vi "DSB Modulation Demo (Baseband-Sine) - Basic.vi"() -> ()   [LabVIEW 2013]
uses:
  <vilib>/express/express analysis/Spectral/Block/exnSpectralBlock spectral measurements power poly.vi
  <vilib>/express/express analysis/Spectral/Block/exnSpectralBlock spectral measurements power DDT.vi
  <vilib>/express/express analysis/Spectral/XNode/ExpressSpectralMeasurementsBlockNode.xnode
panel:
  in  "WAV Sample Rate":dbl=44100.0 caption="dt"
  in  "Modulation Freq.":dbl=2000.0 caption="Frequency"
  in  "LPF Cut-Off":dbl=10000.0 caption="Lower Cut-Off"
  in  "SNR (dB)":dbl(slide)=30.0 caption="Standard deviation" scale=-20.0..30.0
  out "Comparision":dynamicdata(graph)
  out "Baseband":dynamicdata(graph)
  out "DSB FFT":dynamicdata(graph)
  out "DSB Wave":dynamicdata(graph)
  in  "Carrier Amp.":dbl=1.0 caption="Amplitude"
  in  "stop":bool
  in  "Frequency Offset":dbl(slide) scale=0.0..1000.0
  in  "Carrier Freq.":dbl=100000.0 caption="Frequency"
  # "DSB Modulation"
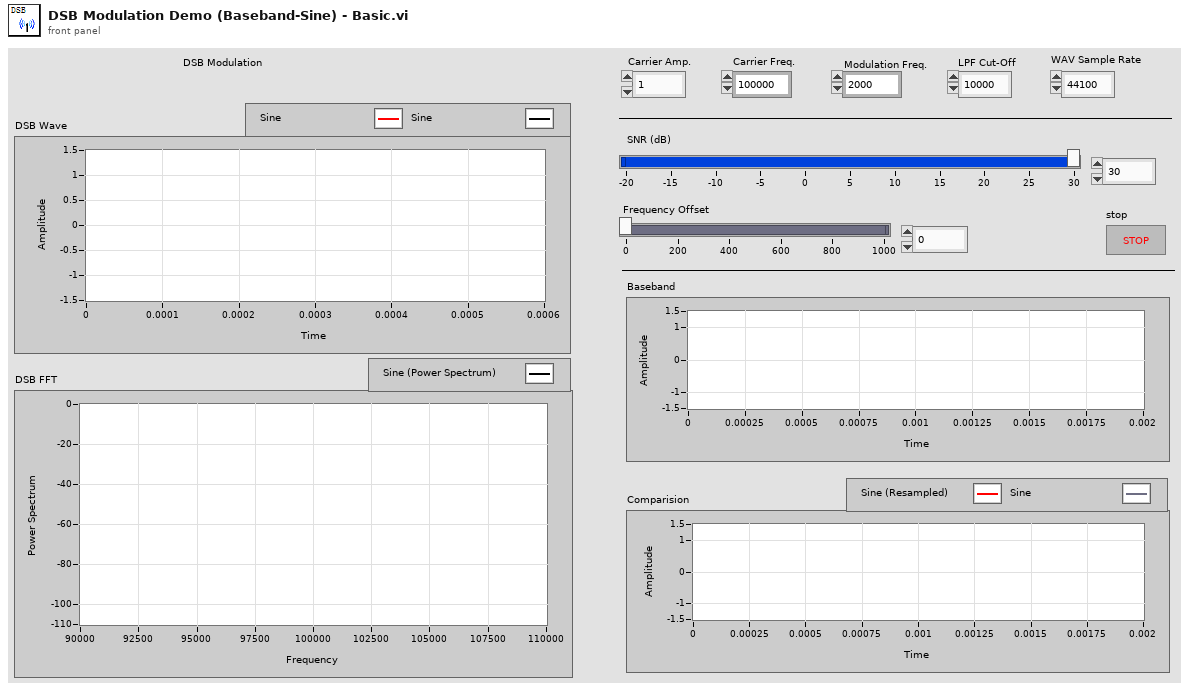
[diagram p1: front panel]
types:
  T1 = cluster{"averaging mode":u16, "weighting mode":u16, "number of averages":u32}
  T2 = cluster{"dB On (F)":bool, "unwrap phase (F)":bool, "convert to degree (F)":bool}
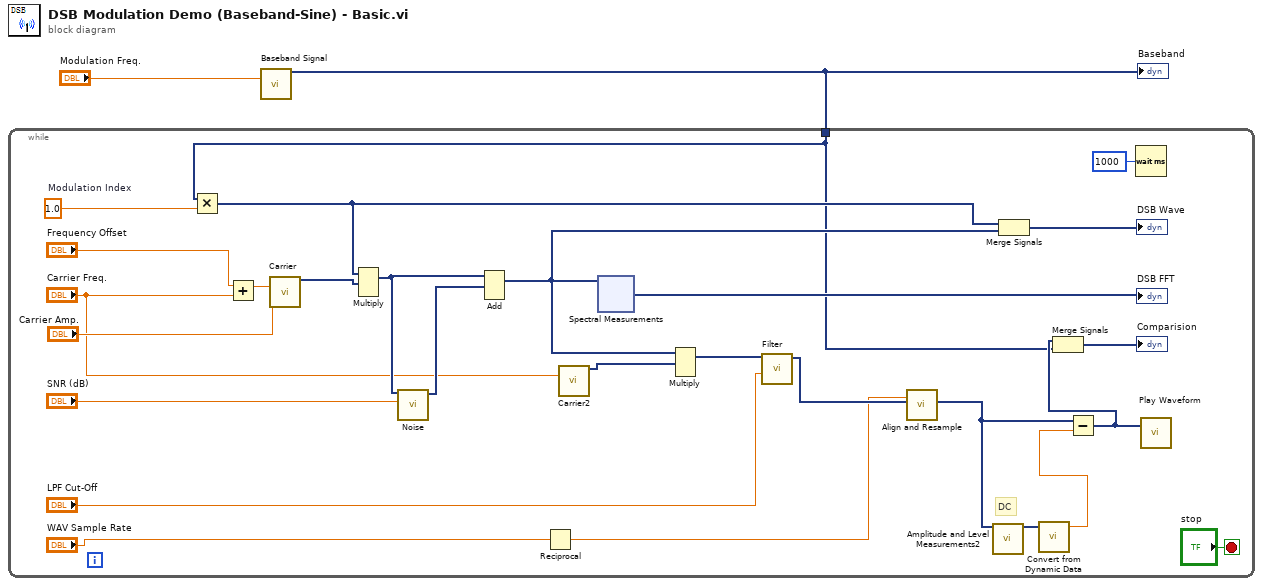
[diagram p0: block diagram]
diagram:
  n1 = call "Baseband Signal"("Frequency"="Modulation Freq.") -> ("Sine"=w1:dynamicdata)  [unwired: 13 in, 1 out]
  "Baseband" <- w1
  n2 = while {
    tunnel: w1 -> [w7]
    stop <- "stop" stop-if-true
    w23 = 1.0  # Modulation Index
    # "DC"
    n3 = Multiply(x=w7, y=w23) -> (x*y=w19:dynamicdata)
    n4 = Add(x="Frequency Offset", y="Carrier Freq.") -> (x+y=w22:dbl)
    n5 = call "Carrier"("Frequency"=w22, "Amplitude"="Carrier Amp.") -> ("Sine"=w20:dynamicdata)  [unwired: 12 in, 1 out]
    n6 = Multiply(1:w20, 2:w19) -> (0:w17:dynamicdata)  [unwired: 1 in, 1 out]
    n7 = call "Noise.vi"("AWGN (dB)"="SNR (dB)", "Dynamic Data"=w17) -> ("DC with Gaussian Noise"=w18:dynamicdata)  [unwired: 9 in]
    n8 = Add(1:w18, 2:w17) -> (0:w12:dynamicdata)  [unwired: 1 in, 1 out]
    n9 = Reciprocal(x="WAV Sample Rate") -> (1/x=w3:dbl)
    n10 = call "Carrier2"("Frequency"="Carrier Freq.") -> ("Sine"=w13:dynamicdata)  [unwired: 13 in, 1 out]
    n11 = xnode "Spectral Measurements"("Signals"=w12) -> ("Power Spectrum"=→"DSB FFT":dynamicdata)  [unwired: 2 in, 2 out]
    n12 = Multiply(1:w13, 2:w12) -> (0:w11:dynamicdata)  [unwired: 1 in, 1 out]
    n13 = call "Filter"("Lower Cut-Off"="LPF Cut-Off", "Signal"=w11) -> ("Filtered Signal"=w10:dynamicdata)  [unwired: 8 in, 1 out]
    n14 = call "Align and Resample"("dt"=w3, "Signals"=w10) -> ("Resampled Signals"=w26:dynamicdata)  [unwired: 7 in, 2 out]
    n15 = call "Amplitude and Level Measurements2"("Signals"=w26) -> ("Mean (DC)"=w28:dynamicdata)  [unwired: 13 in, 1 out]
    n16 = Merge Signals(w19, w12) -> (→"DSB Wave":dynamicdata)
    n17 = call "Convert from Dynamic Data"("Dynamic Data Type"=w28) -> ("Scalar"=w25:dbl)  [unwired: 3 in]
    n18 = Subtract(x=w26, y=w25) -> (x-y=w8:dynamicdata)
    n19 = Merge Signals(w8, w7) -> (→"Comparision":dynamicdata)
    n20 = Wait (ms)(milliseconds to wait=u32 1000) -> ()  [unwired: 1 out]
    n21 = call "Play Waveform"("Data"=w8) -> ()  [unwired: 18 in, 1 out]
  }
